vi "Corridor to End Cube.vi"() -> ()   [LabVIEW 2017]
uses:
  Block Clusters/Corridor to End Cube.ctl
  Support Code/Starting Position.ctl
  <vilib>/Rock Robotics/WPI/Framework/Command Status Info.ctl
  <vilib>/Rock Robotics/WPI/Framework/Completion Status.ctl
  <vilib>/Rock Robotics/WPI/Framework/Completion Notifier.ctl
panel:
  out "Command Info Out":T1
  in  "Starting Position":T4
  in  "Block Inputs":T5
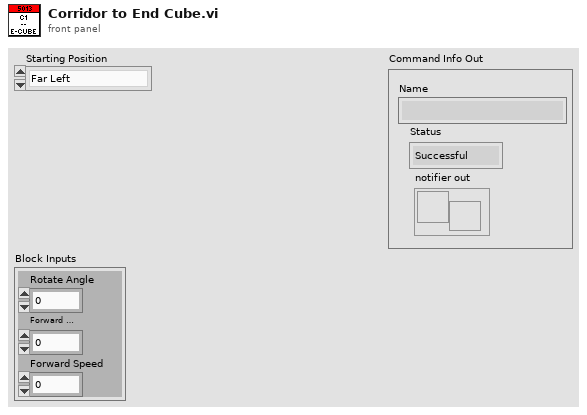
[diagram p1: front panel]
types:
  T1 = typedef "Command Status Info.ctl" = cluster{"Name":string, "Status":T2, "notifier out":T3}
  T2 = typedef "Completion Status.ctl" = enum16{"Successful", "Aborted", "Incomplete"}
  T3 = typedef "Completion Notifier.ctl" = refnum<notifier>
  T4 = typedef "Starting Position.ctl" = enum16{"Far Left", "Center", "Far Right"}
  T5 = typedef "Corridor to End Cube.ctl" = cluster{"Rotate Angle":dbl, "Forward Distance":dbl, "Forward Speed":dbl}
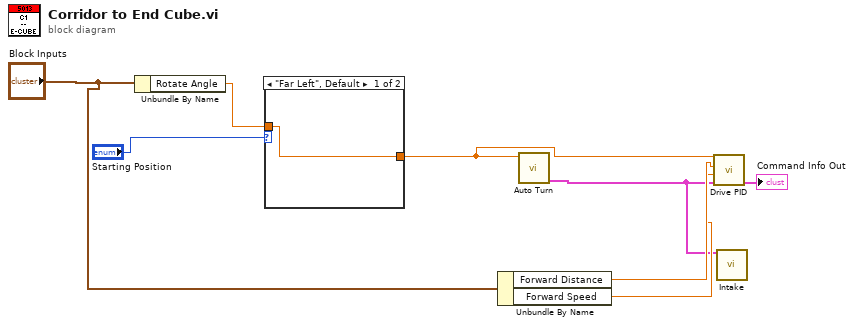
[diagram p0: block diagram]
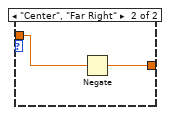
[diagram p2: hidden frame]
diagram:
  n1 = Unbundle By Name("Block Inputs") -> ("Rotate Angle"=w7:dbl)
  n2 = case shown="\"Far Left\", Default" "Starting Position" {
    tunnel: w7 -> [w9 w11]
    tunnel: [w9 w10] -> w5
    frame "Far Left", Default {
    }
    frame "Center", "Far Right" {
      n3 = Negate(x=w11) -> (-x=w10:dbl)
    }
  }
  n4 = Unbundle By Name("Block Inputs") -> ("Forward Distance"=w4:dbl, "Forward Speed"=w3:dbl)
  n5 = call "Auto Turn.vi"("Target Angle"=w5) -> ("Command Info Out"=w1:T1)  [unwired: 10 in]
  n6 = call "Drive PID.vi"("Command Info In"=w1, "Speed"=w3, "Distance"=w4, "Target Angle"=w5) -> ("Command Info Out"=→"Command Info Out":T1)  [unwired: 7 in]
  n7 = call "Intake.vi"("Command Info In"=w1) -> ()  [unwired: 10 in, 1 out]
